vi "Save_Measures_STD_INIT.vi"(8 "appended array":string[](array[string]), 10 "Data in":dbl[][](array[numeric]) format="%0.2f", 11 "file path (dialog if empty)":path) -> ()   [LabVIEW 2012]
uses:
  <vilib>/Utility/file.llb/Write To Spreadsheet File (string).vi
  <vilib>/Utility/file.llb/Write To Spreadsheet File (DBL).vi
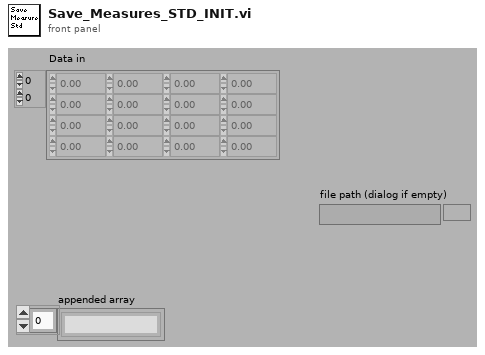
[diagram p1: front panel]
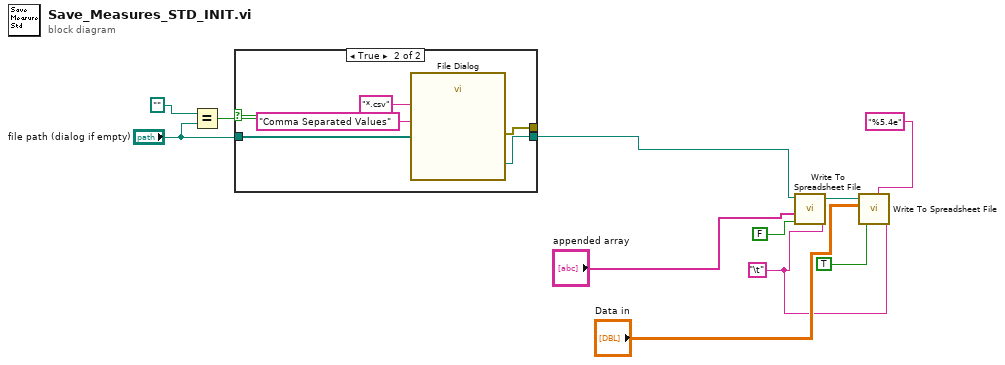
[diagram p0: block diagram]
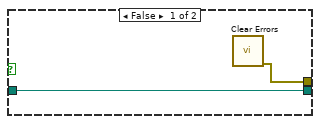
[diagram p2: hidden frame]
diagram:
  w1 = "\t"
  n1 = Equal?(x=path "", y="file path (dialog if empty)") -> (x = y?=w5:bool)
  n2 = case shown="True" w5 {
    tunnel: "file path (dialog if empty)" -> [w13 _]
    tunnel: [w13 w15] -> w2
    tunnel: [w12 w14] -> _
    frame False {
      n3 = call <vilib>:"Clear Errors.vi"() -> ("error out"=w12:errorcluster)  [unwired: 7 in]
    }
    frame True {
      n4 = call "File Dialog"("pattern (all files)"="*.csv", "pattern label"="Comma Separated Values") -> ("selected path"=w15:path, "error out"=w14:errorcluster)  [unwired: 10 in, 2 out]
    }
  }
  n5 = call-poly <vilib>:"Write To Spreadsheet File.vi"("delimiter (\\t)"=w1, "append to file? (new file:F)"=FALSE, "1D data"="appended array", "file path (dialog if empty)"=w2) -> ("new file path (Not A Path if cancelled)"=w9:path)  [unwired: 4 in]
  n6 = call-poly <vilib>:"Write To Spreadsheet File.vi"("delimiter (\\t)"=w1, "format (%.3f)"="%5.4e", "append to file? (new file:F)"=TRUE, "2D data"="Data in", "file path (dialog if empty)"=w9) -> ()  [unwired: 3 in, 1 out]
